vi "Get Provided Interface and Service Class.vi"(8 "error in (no error)":errorcluster, 11 "session factory in":refnum<class "DMM_Base.lvclass">) -> (0 "error out":errorcluster, 1 "service class":string, 2 "provided interface":string, 3 "session factory out":refnum<class "DMM_Base.lvclass">)   [LabVIEW 2021, in "DMM_Base.lvclass"]
uses:
  DMM_Base.lvclass
  DMM_Base.lvclass/DMM_Base.ctl
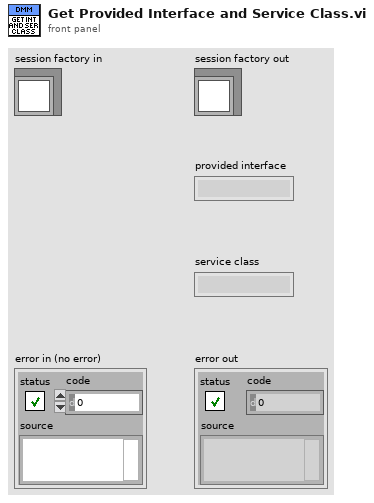
[diagram p1: front panel]
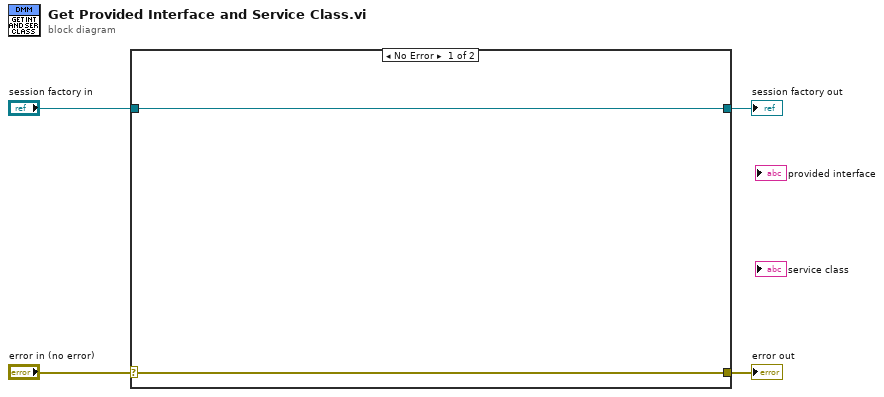
[diagram p0: block diagram]
diagram:
  n1 = case shown="No Error" "error in (no error)" {
    selector: "error in (no error)" -> [w5 w8]
    tunnel: [w5 w8] -> w3
    tunnel: [w6 w7] -> w1
    tunnel: "session factory in" -> [w6 w7]
    frame No Error {
    }
    frame Error {
    }
  }
  "error out" <- w3
  "session factory out" <- w1
